vi "GitImportDir.vi"(7 "VI reference (current VI)":refnum<vi>, 8 "error in (no error)":errorcluster, 9 "Save Repo Path":path=path "", 10 "Import Folder Path":path, 11 "Git exec":string="git") -> (0 "error out":errorcluster, 1 "Repo Path out":path, 2 "Loaded Hashes":string[](array[string]), 3 "Git exec out":string="git", 4 "Number Loaded":i32)   [LabVIEW 2013]
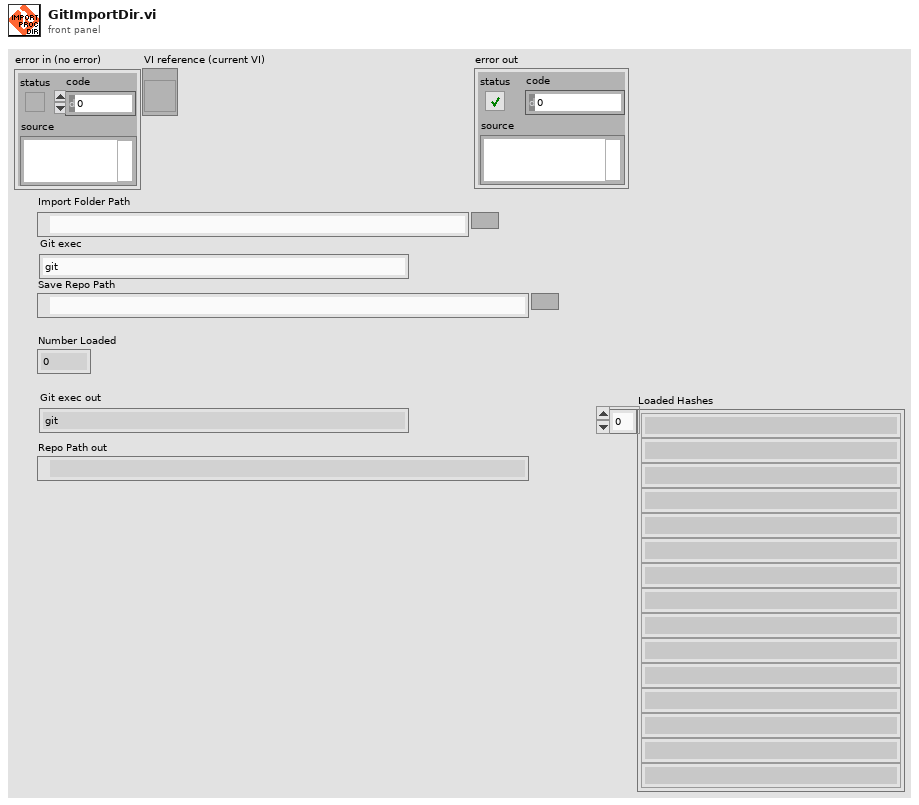
[diagram p1: front panel]
types:
  T1 = cluster{"Title":string, "Description":string, "Author":string}
  T2 = typedef "SaveCluster.ctl" = cluster{"Version":string, "Devices":refnum<class "Device.lvclass">[], "Select Layout":i32, "Layout:Strings And Values []":T3, "User defined functions":string, "VariableManager":refnum<class "VariableManager.lvclass">}
  T3 = typedef "LVStringsAndValuesArrayTypeDef_I32.ctl" = cluster{"String":string, "Value":i32}[]
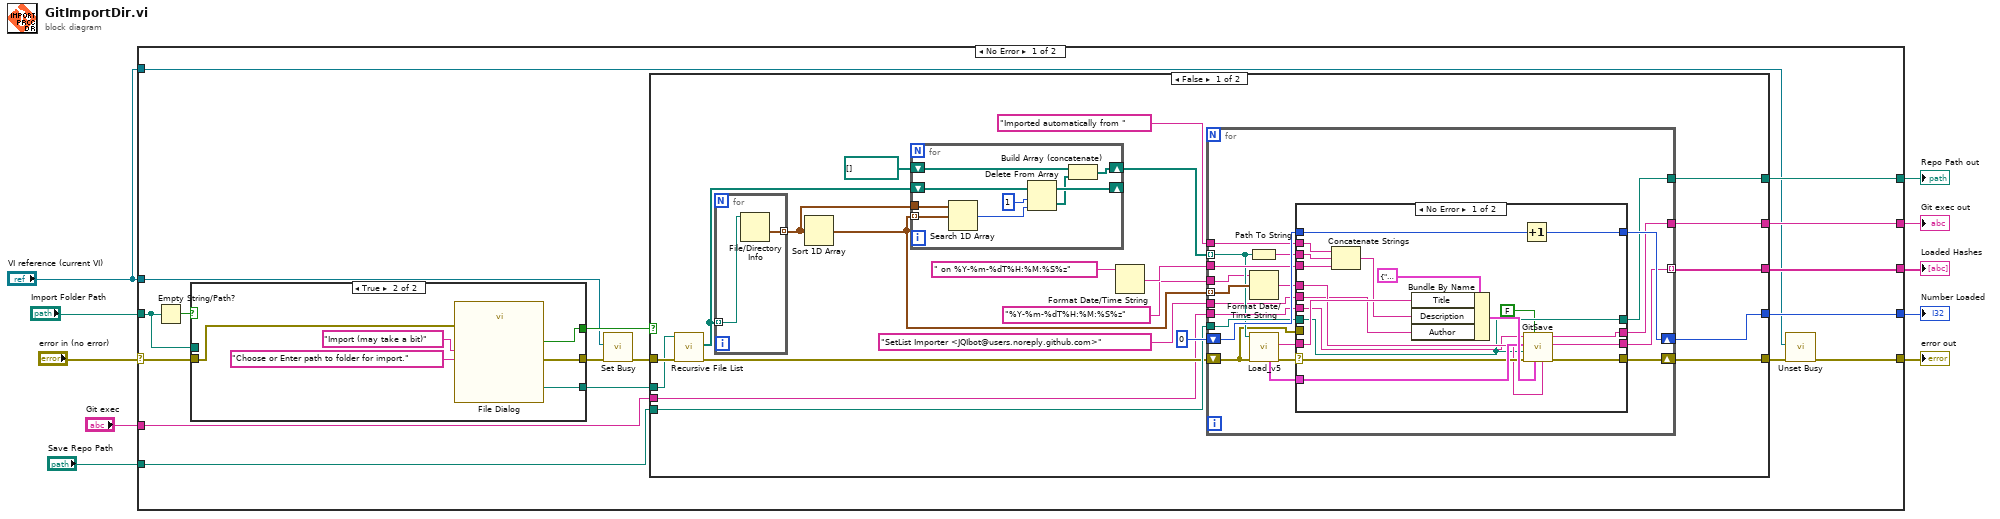
[diagram p0: block diagram]
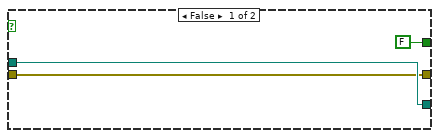
[diagram p2: hidden frame]
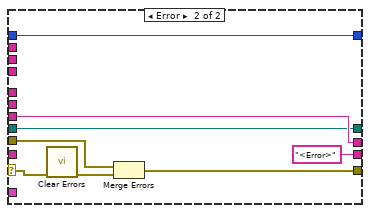
[diagram p3: hidden frame]
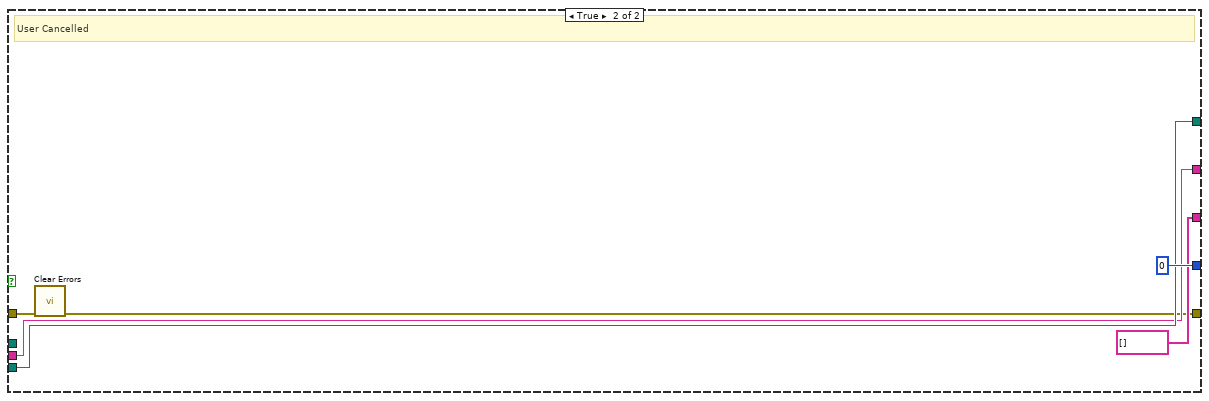
[diagram p4: hidden frame]
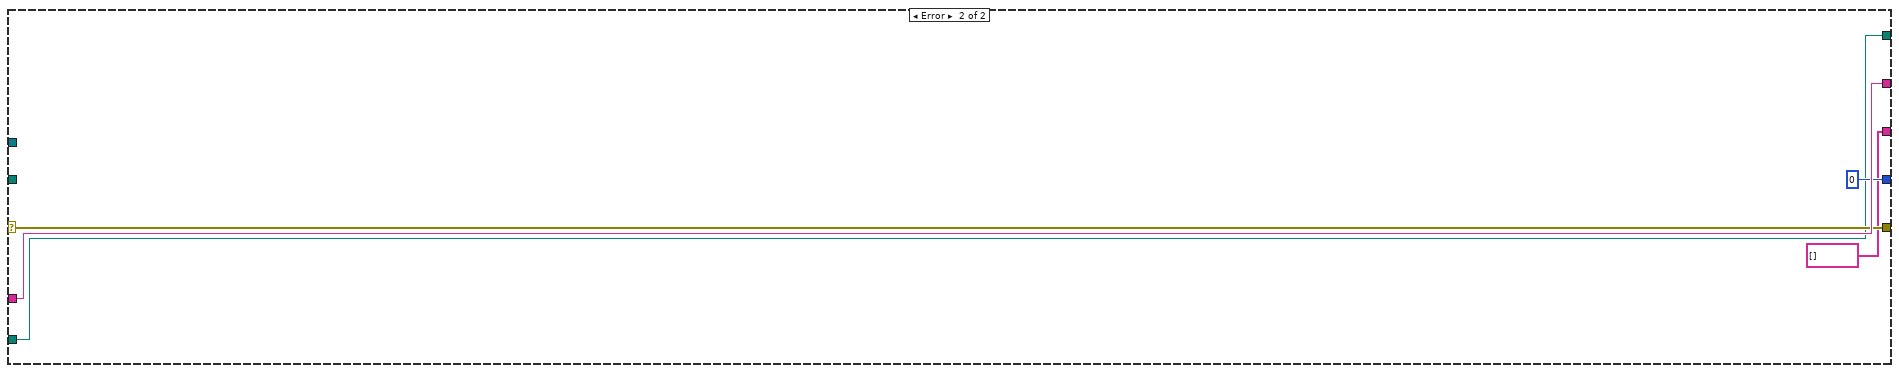
[diagram p5: hidden frame]
diagram:
  n1 = case shown="No Error" "error in (no error)" {
    selector: "error in (no error)" -> [w17 w125]
    tunnel: [w27 string[] []] -> w10
    tunnel: [w26 0] -> w9
    tunnel: "Save Repo Path" -> [w25 w122]
    tunnel: [w24 w126] -> w7
    tunnel: [w13 w125] -> w5
    tunnel: "Git exec" -> [w23 w126]
    tunnel: "Import Folder Path" -> [w19 _]
    tunnel: [w22 w122] -> w2
    tunnel: "VI reference (current VI)" -> [w12 _]
    tunnel: "VI reference (current VI)" -> [w11 _]
    frame No Error {
      n2 = Empty String/Path?(string/path=w19) -> (empty?=w20:bool)
      n3 = case shown="True" w20 {
        tunnel: [FALSE ("cancelled") w36] -> w21
        tunnel: w19 -> [w29 _]
        tunnel: [w29 w35] -> w18
        tunnel: w17 -> [w28 w34]
        tunnel: [w28 w33] -> w16
        frame False {
        }
        frame True {
          n4 = call "File Dialog"("prompt"="Choose or Enter path to folder for import.", "button label"="Import (may take a bit)", "error in"=w34) -> ("selected path"=w35:path, "cancelled"=w36:bool, "error out"=w33:errorcluster)  [unwired: 9 in, 1 out]
        }
      }
      n5 = call <vilib>:"Set Busy.vi"("error in (no error)"=w16, "VI reference (current VI)"=w12) -> ("error out"=w15:errorcluster)  [unwired: 8 in, 1 out]
      n6 = case shown="False" w21 {
        tunnel: [w51 string[] []] -> w27
        tunnel: [w50 0] -> w26
        tunnel: w25 -> [w47 w119]
        tunnel: [w46 w118] -> w24
        tunnel: w15 -> [w45 w117]
        tunnel: [w43 w116] -> w14
        tunnel: w23 -> [w42 w118]
        tunnel: [w41 w119] -> w22
        tunnel: w18 -> [w38 _]
        frame False {
          n7 = call <vilib>:"Recursive File List.vi"("error in (no error)"=w45, "Folder Path"=w38) -> ("error out"=w44:errorcluster, "All Files in Dir"=w56:path[])  [unwired: 5 in, 3 out]
          n8 = for {
            tunnel: w56 -> [w115] mode=indexing
            tunnel: [w114] -> w57 mode=indexing
            n9 = File/Directory Info(path=w115) -> (last mod=w114:timestamp)  [unwired: 1 in, 6 out]
          }
          n10 = Sort 1D Array(array=w57) -> (sorted array=w53:timestamp[])
          n11 = for {
            tunnel: w53 -> [w113] mode=indexing
            tunnel: w57 -> [w112]
            shift-right: [w108] -> _
            shift-left: w56 -> [w111]
            shift-right: [w105] -> w54
            shift-left: path[] [] -> [w106]
            n12 = Search 1D Array(1D array=w112, element=w113) -> (index of element=w110:i32)  [unwired: 1 in]
            n13 = Delete From Array(array=w111, length=1, index=w110) -> (deleted portion=w107:path[], array with subset deleted=w108:path[])
            n14 = Build Array (concatenate)(w106, w107) -> (w105:path[])
          }
          n15 = Format Date/Time String(time format string (%c)=" on %Y-%m-%dT%H:%M:%S%z") -> (date/time string=w49:string)  [unwired: 2 in]
          n16 = for {
            tunnel: w54 -> [w66] mode=indexing
            tunnel: w53 -> [w71] mode=indexing
            shift-right: [w76] -> w50
            shift-left: 0 -> [w75]
            tunnel: [w72] -> w51 mode=indexing
            tunnel: w42 -> [w69]
            tunnel: w47 -> [w68]
            tunnel: w49 -> [w67]
            tunnel: "Imported automatically from " ("time format string (%c)") -> [w64]
            tunnel: [w63] -> w46
            shift-right: [w62] -> w43
            shift-left: w44 -> [w61]
            tunnel: [w60] -> w41
            tunnel: "%Y-%m-%dT%H:%M:%S%z" ("time format string (%c)") -> [w59]
            tunnel: "SetList Importer <JQIbot@users.noreply.github.com>" ("Author") -> [w58]
            n17 = Path To String(path=w66) -> (string=w65:string)
            n18 = Format Date/Time String(time format string (%c)=w59, seconds (now)=w71) -> (date/time string=w70:string)  [unwired: 1 in]
            n19 = call "Load_v5.vi"("error in"=w61, "Path (open dialog)"=w66) -> ("error out"=w77:errorcluster, "Procedure Name"=w74:string, "Save Cluster"=w73:T2)  [unwired: 5 in, 2 out]
            n20 = case shown="No Error" w77 {
              selector: w77 -> [w89 w103]
              tunnel: [w96 w104] -> w76
              tunnel: w75 -> [w95 w104]
              tunnel: w74 -> [w92 _]
              tunnel: w73 -> [w91 _]
              tunnel: [w90 "<Error>" ("Saved Hash")] -> w72
              tunnel: w70 -> [w88 _]
              tunnel: w69 -> [w87 w101]
              tunnel: w68 -> [w80 w97]
              tunnel: w67 -> [w85 _]
              tunnel: w65 -> [w86 _]
              tunnel: w64 -> [w84 _]
              tunnel: [w82 w101] -> w63
              tunnel: [w81 w98] -> w62
              tunnel: w61 -> [_ w100]
              tunnel: [w80 w97] -> w60
              tunnel: w58 -> [w79 _]
              frame No Error {
                n21 = Concatenate Strings(w84, w86, w85) -> (w83:string)
                n22 = Bundle By Name(cluster=T1 {"Title"="", "Description"="", "Author"=""} ("Commit Meta-Info"), "Title"=w92, "Description"=w83, "Author"=w79) -> (w93:T1)
                n23 = Increment(x=w95) -> (x+1=w96:i32)
                n24 = call "GitSave.vi"("Date"=w88, "Commit Meta-Info"=w93, "Make LAST_SAVED"=FALSE, "error in (no error)"=w89, "Save Repo Path"=w80, "Save Cluster"=w91, "Git exec"=w87) -> ("error out"=w81:errorcluster, "Saved Hash"=w90:string, "Git exec out"=w82:string)  [unwired: 1 in, 1 out]
              }
              frame Error {
                n25 = call <vilib>:"Clear Errors.vi"("error in (no error)"=w103) -> ("error out"=w99:errorcluster)  [unwired: 6 in]
                n26 = Merge Errors(w100, w99) -> (w98:errorcluster)
              }
            }
          }
        }
        frame True {
          # "User Cancelled"
          n27 = call <vilib>:"Clear Errors.vi"("error in (no error)"=w117) -> ("error out"=w116:errorcluster)  [unwired: 6 in]
        }
      }
      n28 = call <vilib>:"Unset Busy.vi"("error in (no error)"=w14, "VI reference (current VI)"=w11) -> ("error out"=w13:errorcluster)  [unwired: 9 in]
    }
    frame Error {
    }
  }
  "Loaded Hashes" <- w10
  "Number Loaded" <- w9
  "Repo Path out" <- w2
  "Git exec out" <- w7
  "error out" <- w5
